vi "Trap1-22-05-2017.vi"() -> (4 "U":fxp<+/-,26,5> format="%.23g")   [LabVIEW 2010]
uses:
  <vilib>/eio/EIONode/EIONode.xnode
  <vilib>/rvi/eio/nirviEIOImplementation/nirviEIOImplementation.xnode
  <vilib>/rvi/eio/common/nirviEmuClasses.ctl
  <vilib>/rvi/FXPMathLib/FxpSub/XNode/nifxpmath_Sub.xnode
  <vilib>/rvi/FXPMathLib/FxpSub/subVIs/nifxpmath_Sub_SimConfig.ctl
  <vilib>/fxp/LVFixedPointQuantizationPolicyTypeDef.ctl
  <vilib>/fxp/LVFixedPointOverflowPolicyTypeDef.ctl
  <vilib>/rvi/FXPMathLib/FxpDiv/XNode/nifxpmath_Div.xnode
  <vilib>/rvi/FXPMathLib/FxpDiv/subVIs/nifxpmath_Div_SimConfig.ctl
  <vilib>/rvi/FXPMathLib/FxpAdd/XNode/nifxpmath_Add.xnode
  <vilib>/rvi/FXPMathLib/FxpAdd/subVIs/nifxpmath_Add_SimConfig.ctl
  <vilib>/rvi/FXPMathLib/FxpSqrt/XNode/nifxpmath_Sqrt.xnode
  <vilib>/rvi/FXPMathLib/FxpSqrt/subVIs/nifxpmath_Sqrt_SimConfig.ctl
  <vilib>/rvi/eio/common/nirviEmuTemplateMethod_noerrors.vi
  <vilib>/rvi/FXPMathLib/FxpSub/simVIs/DllFxpSubTemp_sub.vi
  <vilib>/rvi/FXPMathLib/FxpDiv/simVIs/DllFxpDivTemp_sub.vi
  <vilib>/rvi/FXPMathLib/FxpAdd/simVIs/DllFxpAddTemp_sub.vi
  <vilib>/rvi/FXPMathLib/FxpSqrt/simVIs/DllSqrtTemp_sub.vi
panel:
  in  "Rest(ms)":u8
  in  "warten(ms)":u8
  out "T":fxp<+/-,17,11>
  in  "e2":fxp<+/-,28,23>=388706.0
  in  "e1":fxp<+/-,31,21>=-82252.0
  in  "e0":fxp<+/-,20,10>=-25.099609375
  in  "stop":bool
  in  "e3c0":fxp<+/-,22,1>=0.000949859619140625
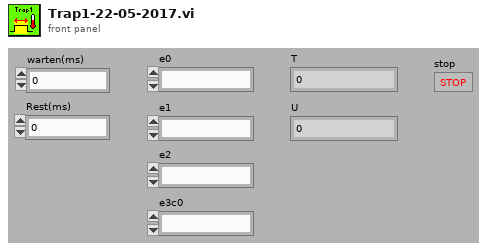
[diagram p1: front panel]
types:
  T1 = typedef "nirviEmuClasses.ctl" = enum16{"IO Read", "IO Write", "Method", "Property Read", "Property Write"}
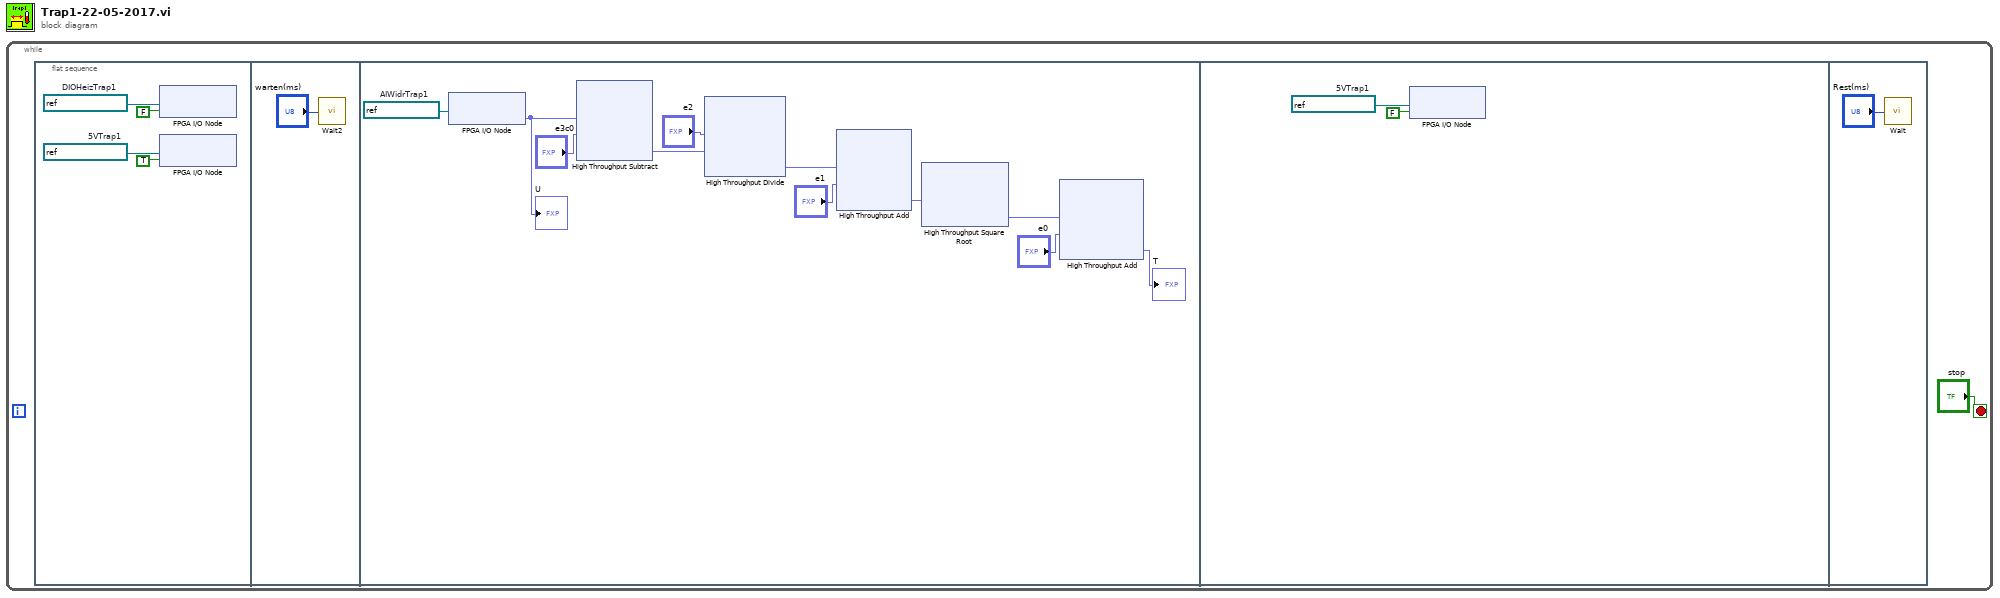
[diagram p0: block diagram]
diagram:
  n1 = while {
    stop <- "stop" stop-if-true
    n2 = flat-sequence {
      frame #0 {
        w3 = refnum<k21> "Mod6/DIO19"  # DIOHeizTrap1
        w5 = refnum<k21> "Mod6/DIO21"  # 5VTrap1
        n3 = xnode "FPGA I/O Node"("I/O Item"=FALSE, "FPGA I/O In"=w3) -> ()  [unwired: 1 out]
        n4 = xnode "FPGA I/O Node"("I/O Item"=TRUE, "FPGA I/O In"=w5) -> ()  [unwired: 1 out]
      }
      frame #1 {
        n5 = call "Wait2"("Count(mSec)"="warten(ms)") -> ()  [unwired: 1 out]
      }
      frame #2 {
        w39 = refnum<k21> "Mod1/AI30"  # AIWidrTrap1
        n6 = xnode "FPGA I/O Node"("FPGA I/O In"=w39) -> ("I/O Item"=w38:fxp<+/-,26,5>)  [unwired: 1 out]
        "U" <- w38
        n7 = xnode "High Throughput Subtract"("x"=w38, "y"="e3c0") -> ("x-y"=w36:fxp<+/-,27,6>)
        n8 = xnode "High Throughput Divide"("x"="e2", "y"=w36) -> ("x/y"=w34:fxp<+/-,44,44>)
        n9 = xnode "High Throughput Add"("x"=w34, "y"="e1") -> ("x+y"=w32:fxp<+,55,45>)
        n10 = xnode "High Throughput Square Root"("x"=w32) -> ("sqrt(x)"=w31:fxp<+,28,23>)
        n11 = xnode "High Throughput Add"("x"=w31, "y"="e0") -> ("x+y"=→"T":fxp<+/-,17,11>)
      }
      frame #3 {
        w196 = refnum<k21> "Mod6/DIO21"  # 5VTrap1
        n12 = xnode "FPGA I/O Node"("I/O Item"=FALSE, "FPGA I/O In"=w196) -> ()  [unwired: 1 out]
      }
      frame #4 {
        n13 = call "Wait"("Count(mSec)"="Rest(ms)") -> ()  [unwired: 1 out]
      }
    }
  }
